vi "set_modifier_base_value.vi"(8 "error in (no error)":errorcluster, 9 "modifier base value":dbl, 10 "modifier index":i32, 11 "GenericTrajectory.lvclass in":refnum<class "TrajectoryDL091126GenericVoxel.lvclass">) -> (0 "error out":errorcluster, 3 "GenericTrajectory.lvclass out":refnum<class "TrajectoryDL091126GenericVoxel.lvclass">)   [LabVIEW 2010, in "TrajectoryDL091126GenericVoxel.lvclass"]
uses:
  TrajectoryDL091126GenericVoxel.lvclass
  TrajectoryDL091126GenericVoxel.lvclass/TrajectoryDL091126GenericVoxel.ctl
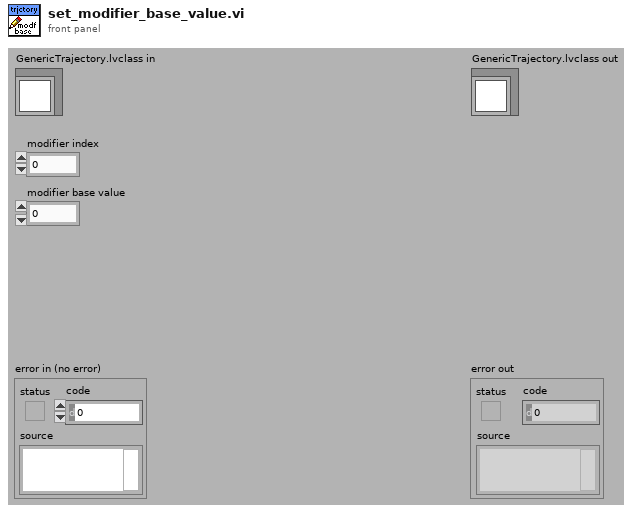
[diagram p1: front panel]
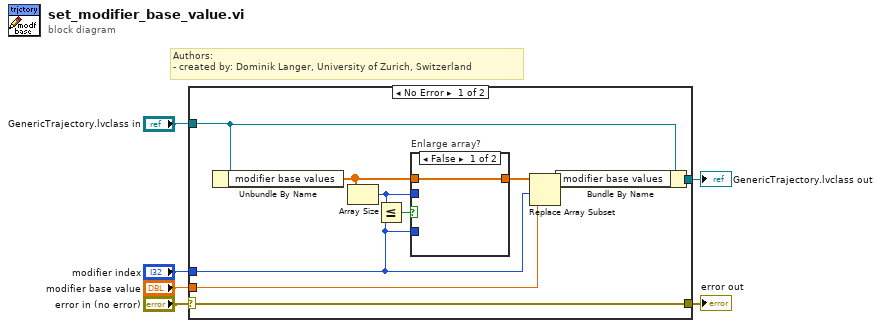
[diagram p0: block diagram]
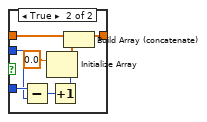
[diagram p2: hidden frame]
diagram:
  # "Authors: \n- created by: Dominik Langer, University of Zurich, Switzerland"
  n1 = case shown="No Error" "error in (no error)" {
    selector: "error in (no error)" -> [w16 w26]
    tunnel: [w16 w26] -> w5
    tunnel: [w15 w27] -> w3
    tunnel: "GenericTrajectory.lvclass in" -> [w14 w27]
    tunnel: "modifier base value" -> [w8 _]
    tunnel: "modifier index" -> [w7 _]
    frame No Error {
      n2 = Unbundle By Name(w14) -> ("modifier base values"=w13:dbl[])
      n3 = Array Size(array=w13) -> (size(s)=w11:i32)
      n4 = Less Or Equal?(x=w11, y=w7) -> (x <= y?=w12:bool)
      n5 = case "Enlarge array?" shown="False" w12 {
        tunnel: w13 -> [w17 w24]
        tunnel: w7 -> [_ w21]
        tunnel: w11 -> [_ w20]
        tunnel: [w17 w25] -> w9
        frame False {
        }
        frame True {
          n6 = Subtract(x=w21, y=w20) -> (x-y=w19:i32)
          n7 = Increment(x=w19) -> (x+1=w18:i32)
          n8 = Initialize Array(0.0 ("element"), w18) -> (w23:dbl[])
          n9 = Build Array (concatenate)(w24, w23) -> (w25:dbl[])
        }
      }
      n10 = Replace Array Subset(array=w9, new element=w8, index=w7) -> (w10:dbl[])
      n11 = Bundle By Name(cluster=w14, "modifier base values"=w10) -> (w15:refnum<class "TrajectoryDL091126GenericVoxel.lvclass">)
    }
    frame Error {
    }
  }
  "error out" <- w5
  "GenericTrajectory.lvclass out" <- w3
